vi "CMN_GetReadoutError.vi"(8 "error in (no error)":errorcluster, 11 "Database RefNum in":T1) -> (0 "error out":errorcluster, 2 "readout_error":errorcluster)   [LabVIEW 2016]
uses:
  DBSHAND/private/vis/DatabaseHand_RefNum.ctl
  DBSHAND/private/vis/DatabaseHand_Element_Get(error).vi
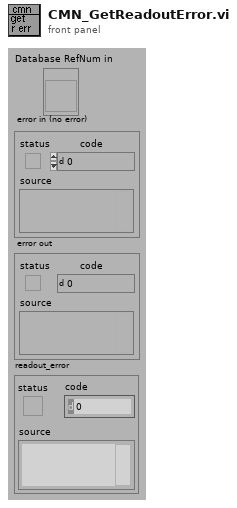
[diagram p1: front panel]
types:
  T1 = typedef "DatabaseHand_RefNum.ctl" = refnum<vi>
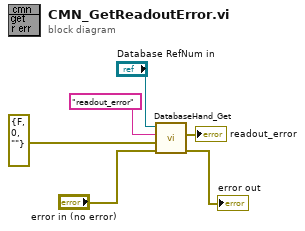
[diagram p0: block diagram]
diagram:
  n1 = call-poly "DatabaseHand_Get.vi"("error in (no error)"="error in (no error)", "default value"=errorcluster {"status"=FALSE, "code"=0, "source"=""} ("error in (no error)"), "name"="readout_error", "Database RefNum in"="Database RefNum in") -> ("error out"=→"error out":errorcluster, "value"=→"readout_error":errorcluster)  [unwired: 1 in, 5 out]
